vi "Close.vi"(8 "error in (no error)":errorcluster, 11 "34972A in":refnum<class "34972A.lvclass">) -> (0 "error out":errorcluster, 3 "34972A out":refnum<class "34972A.lvclass">)   [LabVIEW 2020, in "34972A.lvclass"]
uses:
  34972A.lvclass
  34972A.lvclass/34972A.ctl
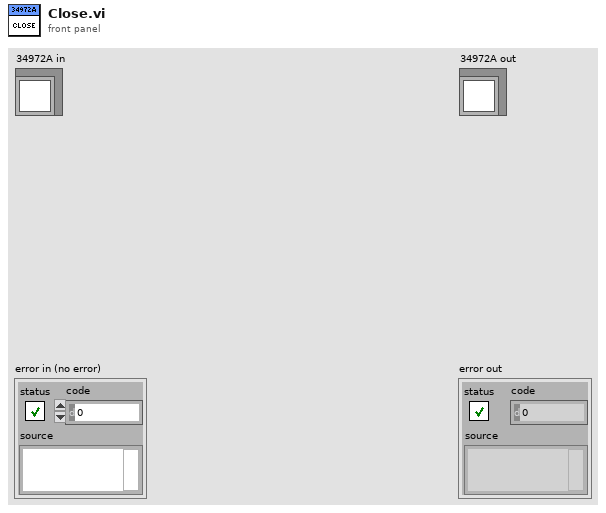
[diagram p1: front panel]
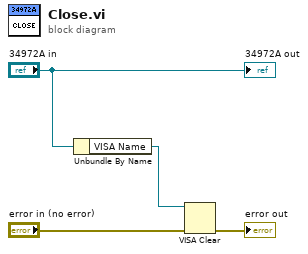
[diagram p0: block diagram]
diagram:
  n1 = Unbundle By Name("34972A in") -> ("VISA Name"=w2:refnum<visa-resource-name>)
  n2 = VISA Clear(VISA resource name=w2, error in (no error)="error in (no error)") -> (error out=→"error out":errorcluster)  [unwired: 1 out]
  "34972A out" <- "34972A in"
